vi "Vertical Toolbar Dialog.vi"(10 "More Options Split Index":i32, 11 "Toolbar Control in":refnum<class "Toolbar Control.lvclass">) -> ()   [LabVIEW 2011, in "Toolbar Control.lvclass"]
doc: "This VI is a dialog VI for the toolbar. When there are too many icons that won't fit into the picture control, a More Options button is shows and clicking it will call this VI, which will be shown at the location of the mouse to display the remaining icons in a vertical list. This VI needs the <B>Toolbar Control in</B> from the previous toolbar, and the <B>More Options Split Index</B> which is the index that the More Options icon is shown at.\n\n-------------\nDeveloped by Brian Hoover (hooovahh)"
uses:
  Toolbar Control.lvclass
  Controls/Horizontal Initialize Settings.ctl
  Controls/Vertical Initialize Settings.ctl
  Non Class Utilities/Show Hide Window Methods.ctl
  Toolbar Control.lvclass/Toolbar Control.ctl
  <vilib>/Utility/miscctls.llb/LVRectTypeDef.ctl
  Controls/Button Pressed User Event Data.ctl
  Controls/Button State.ctl
  Properties/Read Button Pressed Event.vi
  Properties/Read Draw Toolbar Event.vi
  Public Functions/Add Icons From Paths.vi
panel:
  out "2D Picture":picture
  in  "stop":bool
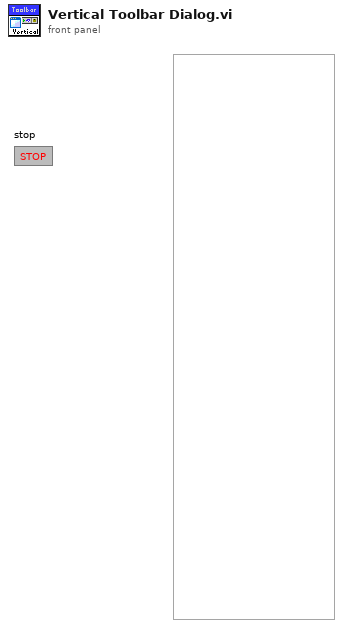
[diagram p1: front panel]
types:
  T1 = typedef "Show Hide Window Methods.ctl" = enum16{"Show Window", "Hide Window", "Close Window", "Minimize Window", "Maximize Window"}
  T2 = typedef "Vertical Initialize Settings.ctl" = cluster{"Button Width":i32, "Button Height":i32, "Separator Height":i32}
  T3 = typedef "Horizontal Initialize Settings.ctl" = cluster{"Button Width":i32, "Button Height":i32, "Separator Width":i32, "More Options Width":i32}
  T4 = typedef "LVRectTypeDef.ctl" = cluster{"left":i16, "top":i16, "right":i16, "bottom":i16}
  T5 = typedef "Toolbar Control.lvclass/Icon Data.ctl" = cluster{"Original Image Path":path, "Original Image Data":T6, "Scaled Icon":picture, "Button Name":string, "Button State":T7, "Icon Type":T8}
  T6 = typedef "imagedata.ctl" = cluster{"image type":i32, "image depth":i32, "image":u8[], "mask":u8[], "colors":u32[], "Rectangle":cluster{"left":i16, "top":i16, "right":i16, "bottom":i16}}
  T7 = typedef "Toolbar Control.lvclass/Button State.ctl" = enum8{"Enabled", "Disabled", "Disabled and Grayed Out"}
  T8 = typedef "Icon Type.ctl" = enum16{"Normal Icon", "Separator Icon", "More Options"}
  T9 = cluster{"left":i16, "top":i16, "right":i16, "bottom":i16}
  T10 = typedef "LVBoundsTypeDef.ctl" = cluster{"Width":u32, "Height":u32}
  T11 = typedef "Button Pressed User Event Data.ctl" = cluster{"Button Pressed":string, "Button State":T7, "Icon Index Over":i32}
  T12 = typedef "LVPoint32TypeDef.ctl" = cluster{"Horizontal":i32, "Vertical":i32}
  T13 = typedef "Button State.ctl" = enum8{"Enabled", "Disabled", "Disabled and Grayed Out"}
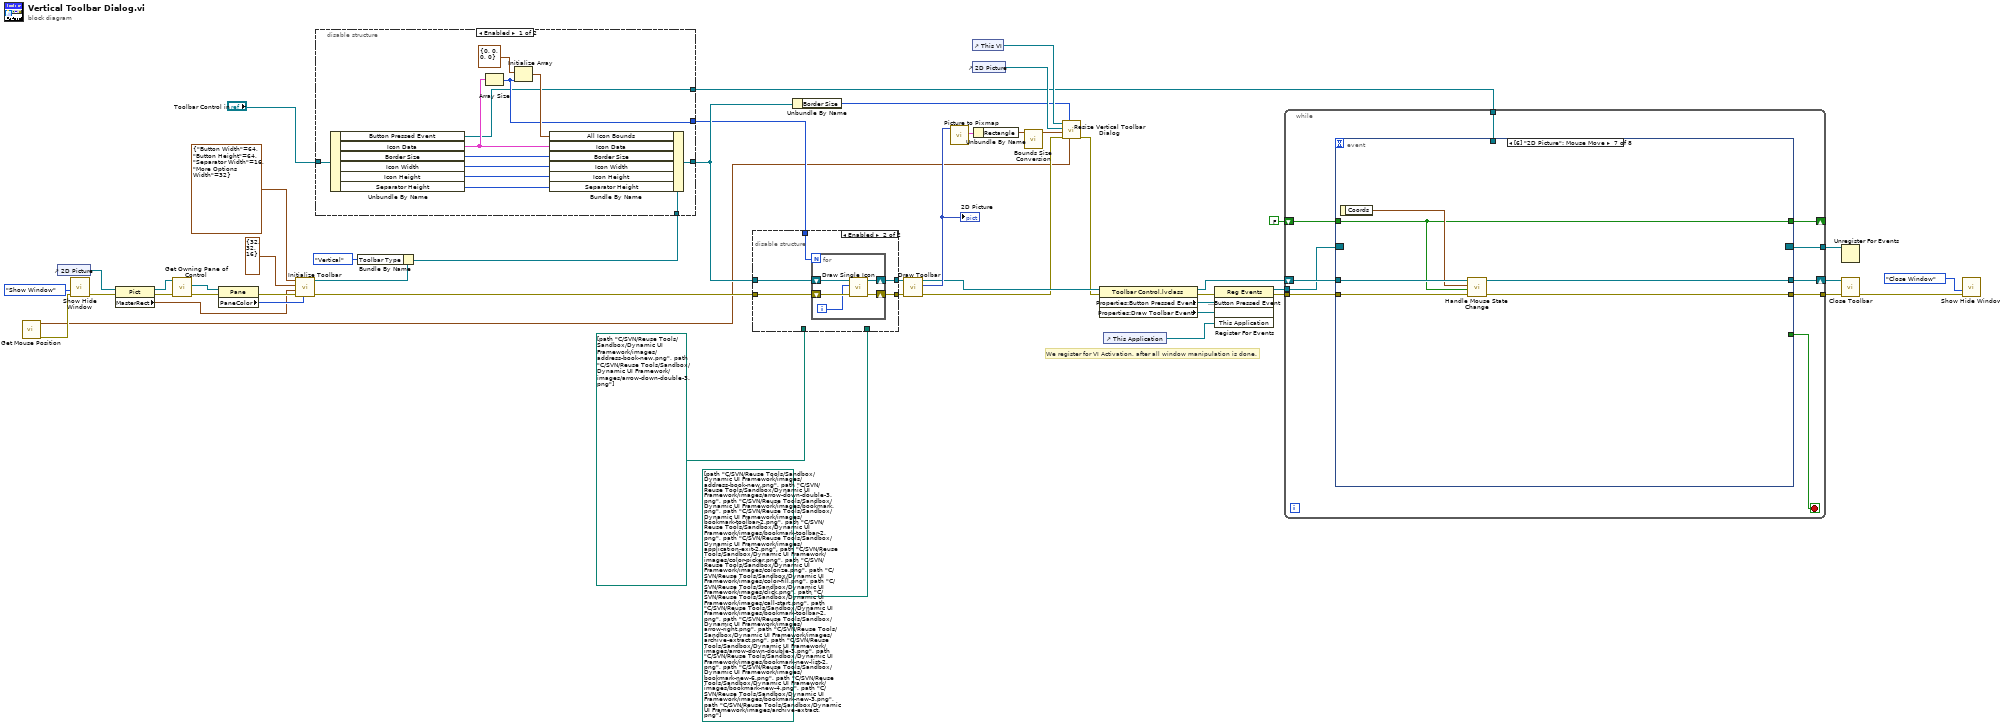
[diagram p0: block diagram]
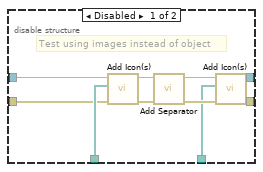
[diagram p2: hidden frame]
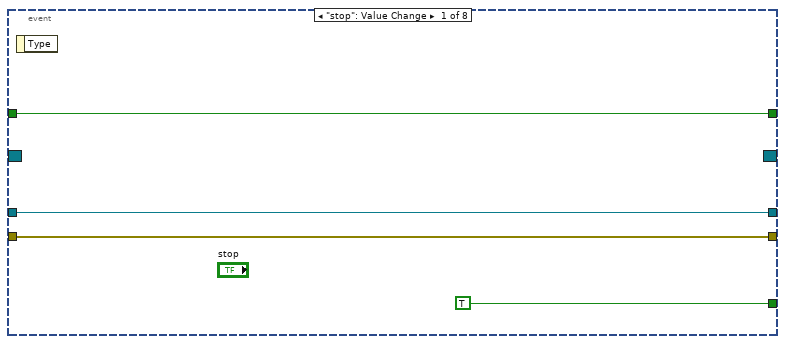
[diagram p4: hidden frame]
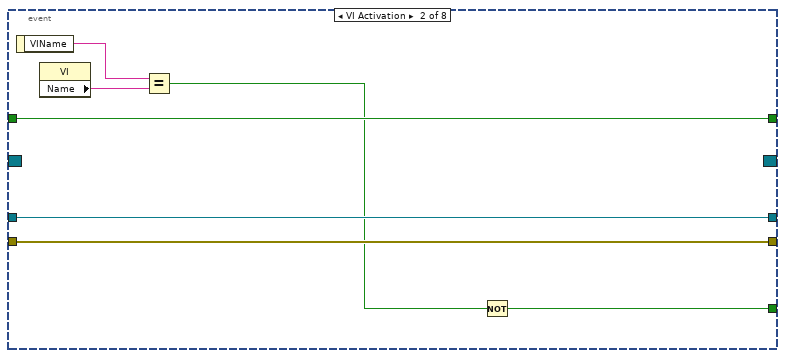
[diagram p5: hidden frame]
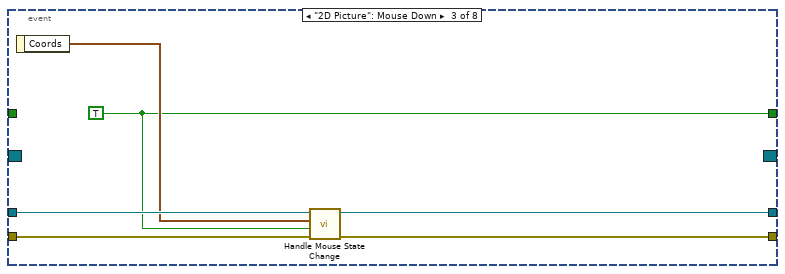
[diagram p6: hidden frame]
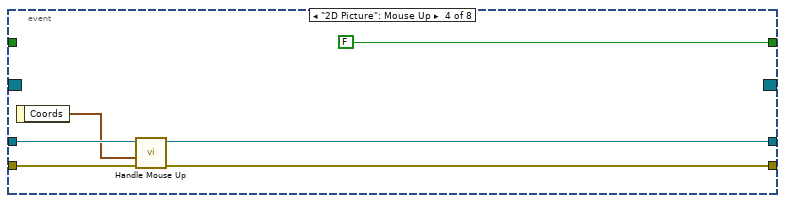
[diagram p7: hidden frame]
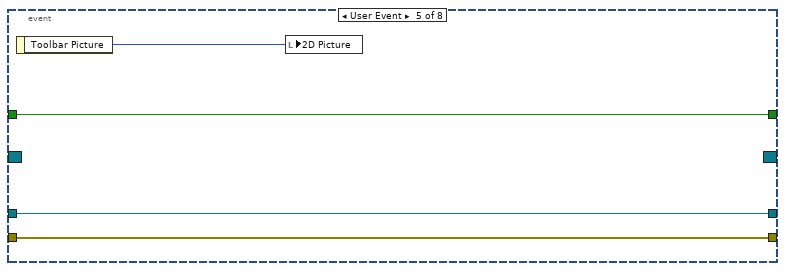
[diagram p8: hidden frame]
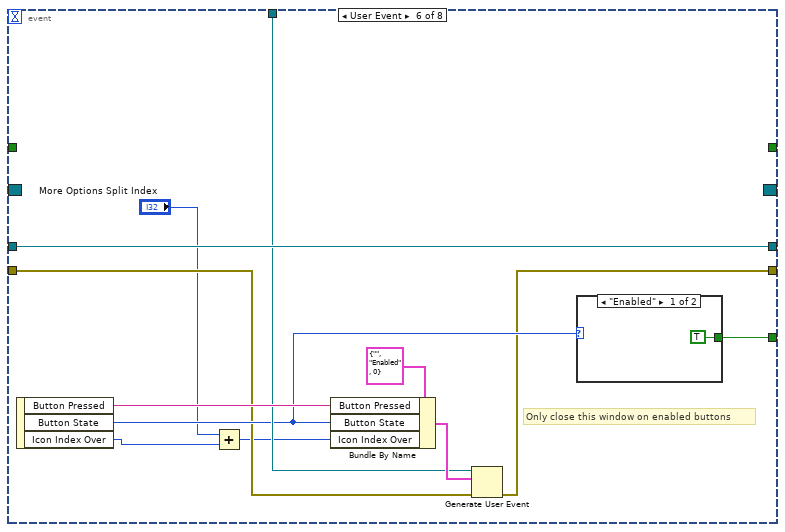
[diagram p9: hidden frame]
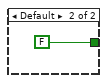
[diagram p10: hidden frame]
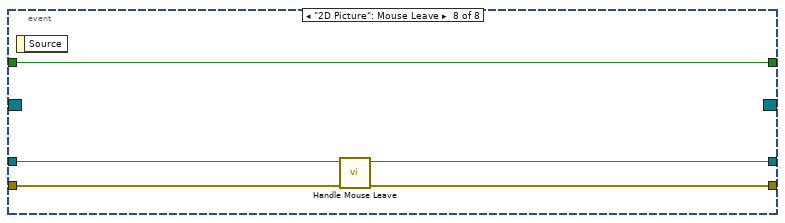
[diagram p11: hidden frame]
diagram:
  # "We register for VI Activation, after all window manipulation is done."
  n1 = call "Get Mouse Position.vi"() -> ("error out"=w4:errorcluster, "Mouse Position"=w3:cluster{"Horizontal":i32, "Vertical":i32})  [unwired: 10 in]
  n2 = control-ref of="2D Picture"() -> (w22:refnum<vi>)
  n3 = call "Show Hide Window.vi"("error in (no error)"=w4, "Method (Show Window)"=Show_Hide_Window_Methods."Show Window") -> ("error out"=w14:errorcluster)  [unwired: 8 in, 1 out]
  n4 = property on="Property Node" class="Pict"(reference=w22, error in=w14) -> (reference out=w47:refnum<vi>, error out=w45:errorcluster, "MasterRect"=w42:T4)
  n5 = call "Get Owning Pane of Control.vi"("error in (no error)"=w45, "Control Refnum"=w47) -> ("error out"=w44:errorcluster, "Owning Pane"=w46:refnum<vi>)  [unwired: 7 in, 1 out]
  n6 = property class="Pane"(reference=w46, error in=w44) -> (error out=w43:errorcluster, "PaneColor"=w48:u32)  [unwired: 1 out]
  n7 = call "Initialize Toolbar.vi"("Background Color"=w48, "error in (no error)"=w43, "Picture Control Bounds"=w42, "Vertical Icon Settings"=T2 {"Button Width"=32, "Button Height"=32, "Separator Height"=16}, "Horizontal Icon Settings"=T3 {"Button Width"=64, "Button Height"=64, "Separator Width"=16, "More Options Width"=32}) -> ("error out"=w27:errorcluster, "Toolbar Control out"=w15:refnum<class "Toolbar Control.lvclass">)  [unwired: 5 in]
  n8 = Bundle By Name(cluster=w15, "Toolbar Type"=enum16{"Horizontal", "Vertical"}."Vertical") -> (w12:refnum<class "Toolbar Control.lvclass">)
  n9 = disable-structure shown="Enabled" {
    disable-tunnel: "Toolbar Control in" -> [w58 _]
    disable-tunnel: w12 -> [w56 w62]
    disable-tunnel: [w55 w62] -> w16
    disable-tunnel: [w51 _] -> w13
    disable-tunnel: [w50 _] -> w9
    frame Enabled {
      n10 = Unbundle By Name(w58) -> ("Button Pressed Event"=w50:refnum<user-event>, "Icon Data"=w54:T5[], "Border Size"=w57:i16, "Icon Width"=w61:i32, "Icon Height"=w60:i32, "Separator Height"=w59:i32)
      n11 = Array Size(array=w54) -> (size(s)=w51:i32)
      n12 = Initialize Array(T4 {"Left"=0, "Top"=0, "Right"=0, "Bottom"=0} ("Icon Bounds"), w51) -> (w52:T4[])
      n13 = Bundle By Name(cluster=w56, "All Icon Bounds"=w52, "Icon Data"=w54, "Border Size"=w57, "Icon Width"=w61, "Icon Height"=w60, "Separator Height"=w59) -> (w55:refnum<class "Toolbar Control.lvclass">)
    }
    frame Disabled {
      # "Test using images instead of object"
    }
  }
  n14 = disable-structure shown="Enabled" {
    disable-tunnel: path[] [path "C:/SVN/Reuse Tools/Sandbox/Dynamic UI Framework/images/address-book-new.png", path "C:/SVN/Reuse Tools/Sandbox/Dynamic UI Framework/images/arrow-down-double-3.png"] -> [w71 _]
    disable-tunnel: [w68 w75] -> w40
    disable-tunnel: [w66 w74] -> w39
    disable-tunnel: path[] [path "C:/SVN/Reuse Tools/Sandbox/Dynamic UI Framework/images/address-book-new.png", path "C:/SVN/Reuse Tools/Sandbox/Dynamic UI Framework/images/arrow-down-double-3.png", path "C:/SVN/Reuse Tools/Sandbox/Dynamic UI Framework/images/bookmark.png", path "C:/SVN/Reuse Tools/Sandbox/Dynamic UI Framework/images/bookmark-toolbar-2.png", path "C:/SVN/Reuse Tools/Sandbox/Dynamic UI Framework/images/bookmark-toolbar-2.png", path "C:/SVN/Reuse Tools/Sandbox/Dynamic UI Framework/images/application-exit-2.png", path "C:/SVN/Reuse Tools/Sandbox/Dynamic UI Framework/images/color-picker.png", path "C:/SVN/Reuse Tools/Sandbox/Dynamic UI Framework/images/colorize.png", path "C:/SVN/Reuse Tools/Sandbox/Dynamic UI Framework/images/color-fill.png", path "C:/SVN/Reuse Tools/Sandbox/Dynamic UI Framework/images/click.png", path "C:/SVN/Reuse Tools/Sandbox/Dynamic UI Framework/images/call-start.png", path "C:/SVN/Reuse Tools/Sandbox/Dynamic UI Framework/images/bookmark-toolbar-2.png", path "C:/SVN/Reuse Tools/Sandbox/Dynamic UI Framework/images/arrow-right.png", path "C:/SVN/Reuse Tools/Sandbox/Dynamic UI Framework/images/archive-extract.png", path "C:/SVN/Reuse Tools/Sandbox/Dynamic UI Framework/images/arrow-down-double-3.png", path "C:/SVN/Reuse Tools/Sandbox/Dynamic UI Framework/images/bookmark-new-list-2.png", path "C:/SVN/Reuse Tools/Sandbox/Dynamic UI Framework/images/bookmark-new-6.png", path "C:/SVN/Reuse Tools/Sandbox/Dynamic UI Framework/images/bookmark-new-4.png", path "C:/SVN/Reuse Tools/Sandbox/Dynamic UI Framework/images/bookmark-new-3.png", path "C:/SVN/Reuse Tools/Sandbox/Dynamic UI Framework/images/archive-extract.png"] -> [w65 _]
    disable-tunnel: w27 -> [w64 w76]
    disable-tunnel: w16 -> [w63 w77]
    disable-tunnel: w13 -> [_ w73]
    frame Disabled {
      # "Test using images instead of object"
      n15 = call-poly "Add Icon(s).vi"("error in (no error)"=w64, "Paths"=w71, "Toolbar Control in"=w63) -> ("error out"=w72:errorcluster, "Toolbar Control out"=w69:refnum<class "Toolbar Control.lvclass">)  [unwired: 7 in]
      n16 = call "Add Separator.vi"("error in (no error)"=w72, "Toolbar Control in"=w69) -> ("error out"=w70:errorcluster, "Toolbar Control out"=w67:refnum<class "Toolbar Control.lvclass">)  [unwired: 8 in]
      n17 = call-poly "Add Icon(s).vi"("error in (no error)"=w70, "Paths"=w65, "Toolbar Control in"=w67) -> ("error out"=w68:errorcluster, "Toolbar Control out"=w66:refnum<class "Toolbar Control.lvclass">)  [unwired: 7 in]
    }
    frame Enabled {
      n18 = for {
        N: w73 -> [_]
        shift-right: [w79] -> w74
        shift-left: w77 -> [w82]
        shift-right: [w80] -> w75
        shift-left: w76 -> [w81]
        i -> [w78]
        n19 = call "Draw Single Icon.vi"("error in (no error)"=w81, "Icon Index"=w78, "Toolbar Control in"=w82) -> ("error out"=w80:errorcluster, "Toolbar Control out"=w79:refnum<class "Toolbar Control.lvclass">)  [unwired: 7 in]
      }
    }
  }
  n20 = Unbundle By Name(w16) -> ("Border Size"=w19:i16)
  n21 = call "Draw Toolbar.vi"("error in (no error)"=w40, "Toolbar Control in"=w39) -> ("error out"=w6:errorcluster, "Toolbar Image"=w23:picture, "Toolbar Control out"=w11:refnum<class "Toolbar Control.lvclass">)  [unwired: 7 in]
  "2D Picture" <- w23
  n22 = call <vilib>:"Picture to Pixmap.vi"("picture"=w23) -> ("image data"=w25:T6)  [unwired: 9 in, 1 out]
  n23 = control-ref of="This VI"() -> (w20:refnum<vi>)
  n24 = control-ref of="2D Picture"() -> (w21:refnum<vi>)
  n25 = Unbundle By Name(w25) -> ("Rectangle"=w24:T9)
  n26 = call "Bounds Size Conversion.vi"("Bounds"=w24) -> ("Size Out"=w18:T10)  [unwired: 9 in, 1 out]
  n27 = call "Resize Vertical Toolbar Dialog.vi"("Mouse Position"=w3, "Border Size"=w19, "error in (no error)"=w6, "Draw Area Size"=w18, "2D Picture Ref"=w21, "Dialog VI Ref"=w20) -> ("error out"=w5:errorcluster)  [unwired: 5 in]
  n28 = property class="Toolbar Control.lvclass"(reference=w11, error in=w5) -> (reference out=w10:refnum<class "Toolbar Control.lvclass">, error out=w37:errorcluster, "Properties:Button Pressed Event"=w35:refnum<user-event>, "Properties:Draw Toolbar Event"=w34:refnum<user-event>)
  n29 = control-ref of="This Application"() -> (w7:refnum<vi>)
  n30 = register-events(error in=w37, w35, w34, w7) -> (reference out=w33:refnum<event-registration>, error out=w36:errorcluster)  [unwired: 1 in]
  n31 = while {
    tunnel: w36 -> [w91]
    shift-right: [w89] -> _
    shift-left: FALSE -> [w90]
    shift-right: [w87] -> w31
    shift-left: w10 -> [w88]
    tunnel: w33 -> [w86]
    tunnel: [w85] -> w32
    tunnel: [w84] -> w30
    tunnel: w9 -> [w83]
    stop <- w92 stop-if-true
    n32 = event shown="[6] \"2D Picture\": Mouse Move" {
      selector: w86 -> [_ _ _ _ _ _ _ _]
      dyn-events: [_ _ _ _ _ _ _ _] -> w85
      timeout: _ -> [_ _ _ _ _ _ _ _]
      tunnel: [TRUE w97 _ _ _ w125 _ _] -> w92
      tunnel: w88 -> [w93 w103 w109 w113 w119 w131 w139 w144]
      tunnel: w91 -> [w94 w102 w108 w112 w118 w123 w138 w143]
      tunnel: w90 -> [w95 w101 _ _ w117 _ w136 w141]
      tunnel: [w95 w101 w106 FALSE w117 _ w136 w141] -> w89
      tunnel: [w94 w102 w105 w114 w118 w122 w135 w142] -> w84
      tunnel: [w93 w103 w104 w110 w119 w131 w134 w140] -> w87
      tunnel: w83 -> [_ _ _ _ _ w126 _ _]
      event "stop": Value Change {
        n33 = event-data() -> ()  [unwired: 1 in, 1 out]
      }
      event VI Activation {
        n34 = event-data() -> ("VIName"=w98:string)  [unwired: 1 in]
        n35 = property class="VI"() -> ("Name"=w99:string)  [unwired: 2 in, 2 out]
        n36 = Equal?(x=w98, y=w99) -> (x = y?=w100:bool)
        n37 = Not(x=w100) -> (.not. x?=w97:bool)
      }
      event "2D Picture": Mouse Down {
        w106 = TRUE
        n38 = event-data() -> ("Coords"=w107:T12)  [unwired: 1 in]
        n39 = call "Handle Mouse State Change.vi"("error in (no error)"=w108, "Mouse Down"=w106, "Mouse Coordinates"=w107, "Toolbar Control in"=w109) -> ("error out"=w105:errorcluster, "Toolbar Control out"=w104:refnum<class "Toolbar Control.lvclass">)  [unwired: 4 in, 2 out]
      }
      event "2D Picture": Mouse Up {
        n40 = event-data() -> ("Coords"=w111:T12)  [unwired: 1 in]
        n41 = call "Handle Mouse Up.vi"("error in (no error)"=w112, "Mouse Coordinates"=w111, "Toolbar Control in"=w113) -> ("error out"=w114:errorcluster, "Toolbar Control out"=w110:refnum<class "Toolbar Control.lvclass">)  [unwired: 4 in, 3 out]
      }
      event User Event {
        n42 = event-data() -> ("Toolbar Picture"=w116:picture)  [unwired: 1 in]
        n43 = local write "2D Picture"(w116) -> ()
      }
      event User Event {
        # "Only close this window on enabled buttons"
        n44 = event-data() -> ("Button Pressed"=w128:string, "Button State"=w124:T13, "Icon Index Over"=w127:i32)  [unwired: 1 in]
        n45 = Add(x="More Options Split Index", y=w127) -> (x+y=w121:i32)
        n46 = Bundle By Name(cluster=T11 {"Button Pressed"="", "Button State"=enum."Enabled", "Icon Index Over"=0} ("Button Pressed"), "Button Pressed"=w128, "Button State"=w124, "Icon Index Over"=w121) -> (w129:T11)
        n47 = Generate User Event(user event=w126, event data cluster=w129, error in=w123) -> (error out=w122:errorcluster)  [unwired: 1 out]
        n48 = case shown="\"Enabled\"" w124 {
          tunnel: [TRUE FALSE] -> w125
          frame "Enabled" {
          }
          frame Default {
          }
        }
      }
      event "2D Picture": Mouse Move {
        n49 = event-data() -> ("Coords"=w137:T12)  [unwired: 1 in]
        n50 = call "Handle Mouse State Change.vi"("error in (no error)"=w138, "Mouse Down"=w136, "Mouse Coordinates"=w137, "Toolbar Control in"=w139) -> ("error out"=w135:errorcluster, "Toolbar Control out"=w134:refnum<class "Toolbar Control.lvclass">)  [unwired: 4 in, 2 out]
      }
      event "2D Picture": Mouse Leave {
        n51 = event-data() -> ()  [unwired: 1 in, 1 out]
        n52 = call "Handle Mouse Leave.vi"("error in (no error)"=w143, "Toolbar Control in"=w144) -> ("error out"=w142:errorcluster, "Toolbar Control out"=w140:refnum<class "Toolbar Control.lvclass">)  [unwired: 7 in, 1 out]
      }
    }
  }
  n53 = Unregister For Events(event registration refnum=w32) -> ()  [unwired: 1 in, 1 out]
  n54 = call "Close Toolbar.vi"("error in (no error)"=w30, "Toolbar Control in"=w31) -> ("error out"=w8:errorcluster)  [unwired: 9 in]
  n55 = call "Show Hide Window.vi"("error in (no error)"=w8, "Method (Show Window)"=Show_Hide_Window_Methods."Close Window") -> ()  [unwired: 8 in, 2 out]
